vi "SZONE.vi"() -> ()   [LabVIEW 2017]
uses:
  040-typeDefs/Position.ctl
  <vilib>/myRIO/Common/Instrument Driver Framework/myRIO v1.0/Encoder/typedefs/Encoder Signal Mode.ctl
  <vilib>/myRIO/Instrument Drivers/Onboard IO/Encoder/typedefs/Encoder Reference.ctl
  <vilib>/myRIO/Common/Instrument Driver Framework/Utilities/typedefs/myRIO Generic Hardware Reference.ctl
  <vilib>/myRIO/Common/Instrument Driver Framework/Utilities/typedefs/Hardware Version Enum.ctl
  <vilib>/myRIO/Common/Instrument Driver Framework/Utilities/typedefs/myRIO v1.0 Reference.ctl
  <vilib>/myRIO/Common/Instrument Driver Framework/Utilities/typedefs/Generic FPGA Reference.ctl
  <vilib>/myRIO/Common/Instrument Driver Framework/myRIO v1.0/Encoder/typedefs/Encoder Channels Enum.ctl
  <vilib>/myRIO/Common/Instrument Driver Framework/myRIO v1.0/Encoder/typedefs/Encoder Configuration v1.0.ctl
  <vilib>/userdefined/High Color/nirio_resource_hc.ctl
  <vilib>/myRIO/Common/Instrument Driver Framework/Utilities/vis/Is FPGA Ref Available.vi
  <vilib>/myRIO/Common/Instrument Driver Framework/myRIO v1.0/Encoder/vis/myRIO v1.1 Open Encoder.vi
  <vilib>/myRIO/Instrument Drivers/Onboard IO/Encoder/vis/Read.vi
  <vilib>/myRIO/Common/Instrument Driver Framework/Utilities/vis/Validate Channels.vi
  <vilib>/myRIO/Common/Instrument Driver Framework/myRIO v1.0/Encoder/vis/myRIO v1.0 Reserve Encoder.vi
  <vilib>/myRIO/Common/Instrument Driver Framework/myRIO v1.0/Encoder/vis/myRIO v1.0 Build MUX Configuration Encoder.vi
  <vilib>/myRIO/Common/Instrument Driver Framework/myRIO v1.0/Resource Manager/vis/myRIO v1.0 Reserve Channel List.vi
  <vilib>/myRIO/Common/Instrument Driver Framework/myRIO v1.0/Resource Manager/vis/myRIO v1.0 Create Configuration List.vi
  <vilib>/myRIO/Common/Instrument Driver Framework/myRIO v1.0/Resource Manager/vis/myRIO v1.0 Reserve Channel.vi
  <vilib>/myRIO/Common/Instrument Driver Framework/myRIO v1.0/Resource Manager/vis/myRIO v1.0 Unreserve Channel.vi
  <vilib>/myRIO/Common/Instrument Driver Framework/myRIO v1.0/Resource Manager/vis/myRIO v1.0 Build Mutex Name.vi
  <vilib>/Utility/VariantDataType/GetNumericInfo.vi
  <vilib>/Utility/error.llb/Error Cluster From Error Code.vi
  <vilib>/myRIO/Common/Instrument Driver Framework/myRIO v1.0/myRIO v1.1 Open.vi
  <vilib>/myRIO/Common/Instrument Driver Framework/Utilities/vis/IO Manager.vi
  <vilib>/myRIO/Common/Instrument Driver Framework/Utilities/vis/Configuration Manager.vi
  <vilib>/myRIO/Common/Instrument Driver Framework/myRIO v1.0/Resource Manager/vis/myRIO v1.0 Configure IO.vi
  <vilib>/myRIO/Common/Instrument Driver Framework/myRIO v1.0/myRIO v1.0 Close.vi
  <vilib>/myRIO/Common/Instrument Driver Framework/myRIO v1.0/Encoder/vis/myRIO v1.0 Configure Encoder.vi
  <vilib>/myRIO/Common/Instrument Driver Framework/myRIO v1.0/Encoder/vis/myRIO v1.0 Read Encoder.vi
  <vilib>/addons/control/pid/pid.llb/PID (DBL).vi
  <vilib>/myRIO/Express VI/Onboard IO/Encoder/Encoder Express VI.xnode
  <vilib>/myRIO/Instrument Drivers/Onboard IO/Encoder/vis/myRIO Encoder Open.xnode
  <vilib>/myRIO/Common/Instrument Driver Framework/myRIO v1.0/Encoder/typedefs/Encoder Count Direction Enum.ctl
  <vilib>/addons/control/pid/NI_PID_pid.lvlib
  <vilib>/myRIO/Instrument Drivers/Onboard IO/Encoder/Encoder.lvlib
panel:
  in  "Array 5":T1[](array[typedef])=[{"X Pos"=0.0, "Y Pos"=600.0, "Bearing"=0.0}]
  out "Setpoint B 5":dbl(slide)=2.6362825367881695 scale=-10.0..10.0
  out "Setpoint A 5":dbl(slide)=-0.6362825367881695 scale=-10.0..10.0
  out "PID B 5":T2(graph)={"Setpoint"=2.6362825367881695, "output"=0.1428270193177578, "dx/dt"=2.2}
  out "PID A 5":T2(graph)={"Setpoint"=-0.6362825367881695, "output"=-0.0025317711853224956, "dx/dt"=0.0}
  out "OUTPUT A 5":dbl(slide) scale=-10.0..10.0
  out "OUTPUT B 5":dbl(slide)=2.2 scale=-10.0..10.0
  in  "stop 5":bool
  in  "PID gains 5":T3={"proportional gain (Kc)"=0.05, "integral time (Ti, min)"=0.05, "derivative time (Td, min)"=0.0} {"derivative time (Td, min)" format="%.3f"; "integral time (Ti, min)" format="%.3f"; "proportional gain (Kc)" format="%.3f"}
  out "XY Graph 5":cluster{"X":dbl, "Y":dbl}[](graph)=[{"X"=4.58646871556769, "Y"=591.0475853292933}, {"X"=4.6524580319359865, "Y"=591.6424095228513}]
  out "PID Angle 5":cluster{"Bearing":dbl, dbl}(graph)={"Bearing"=-29.103573934109825, 6.330461538461682}
  in  "threshold 5":dbl=10.0
  in  "Max Speed 5":dbl=3.0
  in  "Min Speed 5":dbl=1.0
  out "Final X, Y, BEARING 2":cluster{dbl, dbl, dbl}={4.6524580319359865, 591.6424095228513, 6.330461538461682}
  in  "Array 4":T1[](array[typedef])=[{"X Pos"=0.0, "Y Pos"=400.0, "Bearing"=0.0}]
  out "Setpoint B 4":dbl(slide)=-0.8927738654788293 scale=-10.0..10.0
  out "Setpoint A 4":dbl(slide)=2.892773865478829 scale=-10.0..10.0
  out "PID B 4":T2(graph)={"Setpoint"=-0.8927738654788293, "output"=-0.02661516707895155, "dx/dt"=0.25}
  out "PID A 4":T2(graph)={"Setpoint"=2.892773865478829, "output"=0.16937771953511035, "dx/dt"=1.8520000000000039}
  out "OUTPUT A 4":dbl(slide)=1.8520000000000039 scale=-10.0..10.0
  out "OUTPUT B 4":dbl(slide)=0.25 scale=-10.0..10.0
  in  "stop 4":bool
  in  "PID gains 4":T3={"proportional gain (Kc)"=0.05, "integral time (Ti, min)"=0.05, "derivative time (Td, min)"=0.0} {"derivative time (Td, min)" format="%.3f"; "integral time (Ti, min)" format="%.3f"; "proportional gain (Kc)" format="%.3f"}
  out "XY Graph 4":cluster{"X":dbl, "Y":dbl}[](graph)=[{"X"=1.8269883604661505, "Y"=389.9920566702926}, {"X"=1.4195755255413918, "Y"=390.27970964542567}]
  out "PID Angle 4":cluster{"Bearing":dbl, dbl}(graph)={"Bearing"=-8.308879541892331, -54.77607692307679}
  out "X, Y, BEARING 5":cluster{dbl, dbl, dbl}={1.8269883604661505, 389.9920566702926, -55.01053846153833}
  in  "threshold 4":dbl=10.0
  in  "Max Speed 4":dbl=3.0
  in  "Min Speed 4":dbl=1.0
  in  "Array 3":T1[](array[typedef])=[{"X Pos"=50.0, "Y Pos"=300.0, "Bearing"=0.0}]
  out "Setpoint B 3":dbl(slide)=4.472452663359389 scale=-10.0..10.0
  out "Setpoint A 3":dbl(slide)=-2.4724526633593893 scale=-10.0..10.0
  out "PID B 3":T2(graph)={"Setpoint"=4.472452663359389, "output"=0.25941571832624116, "dx/dt"=2.6666666666666665}
  out "PID A 3":T2(graph)={"Setpoint"=-2.4724526633593893, "output"=-0.12167374508156988, "dx/dt"=-0.617333333333363}
  out "OUTPUT A 3":dbl(slide)=-0.617333333333363 scale=-10.0..10.0
  out "OUTPUT B 3":dbl(slide)=2.6666666666666665 scale=-10.0..10.0
  in  "stop 3":bool
  in  "PID gains 3":T3={"proportional gain (Kc)"=0.05, "integral time (Ti, min)"=0.05, "derivative time (Td, min)"=0.0} {"derivative time (Td, min)" format="%.3f"; "integral time (Ti, min)" format="%.3f"; "proportional gain (Kc)" format="%.3f"}
  out "XY Graph 3":cluster{"X":dbl, "Y":dbl}[](graph)=[{"X"=51.50197299547876, "Y"=290.05042940786}, {"X"=52.04283133633413, "Y"=290.306637655666}]
  out "PID Angle 3":cluster{"Bearing":dbl, dbl}(graph)={"Bearing"=-11.90067630737299, 64.65276923076935}
  out "X, Y, BEARING 4":cluster{dbl, dbl, dbl}={51.50197299547876, 290.05042940786, 65.2389230769232}
  in  "threshold 3":dbl=10.0
  in  "Max Speed 3":dbl=3.0
  in  "Min Speed 3":dbl=1.0
  out "Final X, Y, BEARING 3":cluster{dbl, dbl, dbl}={52.04283133633413, 290.306637655666, 64.65276923076935}
  in  "Array 2":T1[](array[typedef])=[{"X Pos"=-50.0, "Y Pos"=200.0, "Bearing"=0.0}]
  out "Setpoint B 2":dbl(slide)=-1.015688327057204 scale=-10.0..10.0
  out "Setpoint A 2":dbl(slide)=3.015688327057204 scale=-10.0..10.0
  out "PID B 2":T2(graph)={"Setpoint"=-1.015688327057204, "output"=-0.029047263301404516, "dx/dt"=0.0}
  out "PID A 2":T2(graph)={"Setpoint"=3.015688327057204, "output"=0.17494784648736927, "dx/dt"=2.0372000000000012}
  out "OUTPUT A 2":dbl(slide)=2.0372000000000012 scale=-10.0..10.0
  out "OUTPUT B 2":dbl(slide) scale=-10.0..10.0
  in  "stop 2":bool
  in  "PID gains 2":T3={"proportional gain (Kc)"=0.05, "integral time (Ti, min)"=0.05, "derivative time (Td, min)"=0.0} {"derivative time (Td, min)" format="%.3f"; "integral time (Ti, min)" format="%.3f"; "proportional gain (Kc)" format="%.3f"}
  out "XY Graph 2":cluster{"X":dbl, "Y":dbl}[](graph)=[{"X"=-46.776161789477904, "Y"=190.23411508966225}, {"X"=-47.2659069619301, "Y"=190.48132411696224}]
  out "PID Angle 2":cluster{"Bearing":dbl, dbl}(graph)={"Bearing"=-16.02589683272788, -63.216692307692256}
  out "X, Y, BEARING 3":cluster{dbl, dbl, dbl}={-46.776161789477904, 190.23411508966225, -63.53907692307687}
  in  "threshold 2":dbl=10.0
  in  "Max Speed 2":dbl=3.0
  in  "Min Speed 2":dbl=1.0
  in  "Array":T1[](array[typedef])=[{"X Pos"=50.0, "Y Pos"=100.0, "Bearing"=0.0}]
  out "Setpoint B":dbl(slide)=1.38366799687848 scale=-10.0..10.0
  out "Setpoint A":dbl(slide)=0.61633200312152 scale=-10.0..10.0
  out "PID B":T2(graph)={"Setpoint"=1.38366799687848, "output"=0.09818267680403459, "dx/dt"=1.0}
  out "PID A":T2(graph)={"Setpoint"=0.61633200312152, "output"=0.0467575940181558, "dx/dt"=1.1111999999999624}
  out "OUTPUT A":dbl(slide)=1.1111999999999624 scale=-10.0..10.0
  out "OUTPUT B":dbl(slide)=1.0 scale=-10.0..10.0
  in  "stop":bool
  in  "PID gains":T3={"proportional gain (Kc)"=0.05, "integral time (Ti, min)"=0.05, "derivative time (Td, min)"=0.0} {"derivative time (Td, min)" format="%.3f"; "integral time (Ti, min)" format="%.3f"; "proportional gain (Kc)" format="%.3f"}
  out "XY Graph":cluster{"X":dbl, "Y":dbl}[](graph)=[{"X"=44.78345806896074, "Y"=90.79679866901255}, {"X"=45.16607487440638, "Y"=91.25698862034483}]
  out "PID Angle":cluster{"Bearing":dbl, dbl}(graph)={"Bearing"=28.937774880309213, 39.74123076923079}
  out "X, Y, BEARING 2":cluster{dbl, dbl, dbl}={44.78345806896074, 90.79679866901255, 39.74123076923079}
  in  "threshold":dbl=10.0
  in  "Max Speed":dbl=3.0
  in  "Min Speed":dbl=1.0
  in  "Initial X, Y, BEARING":cluster{dbl, dbl, dbl}
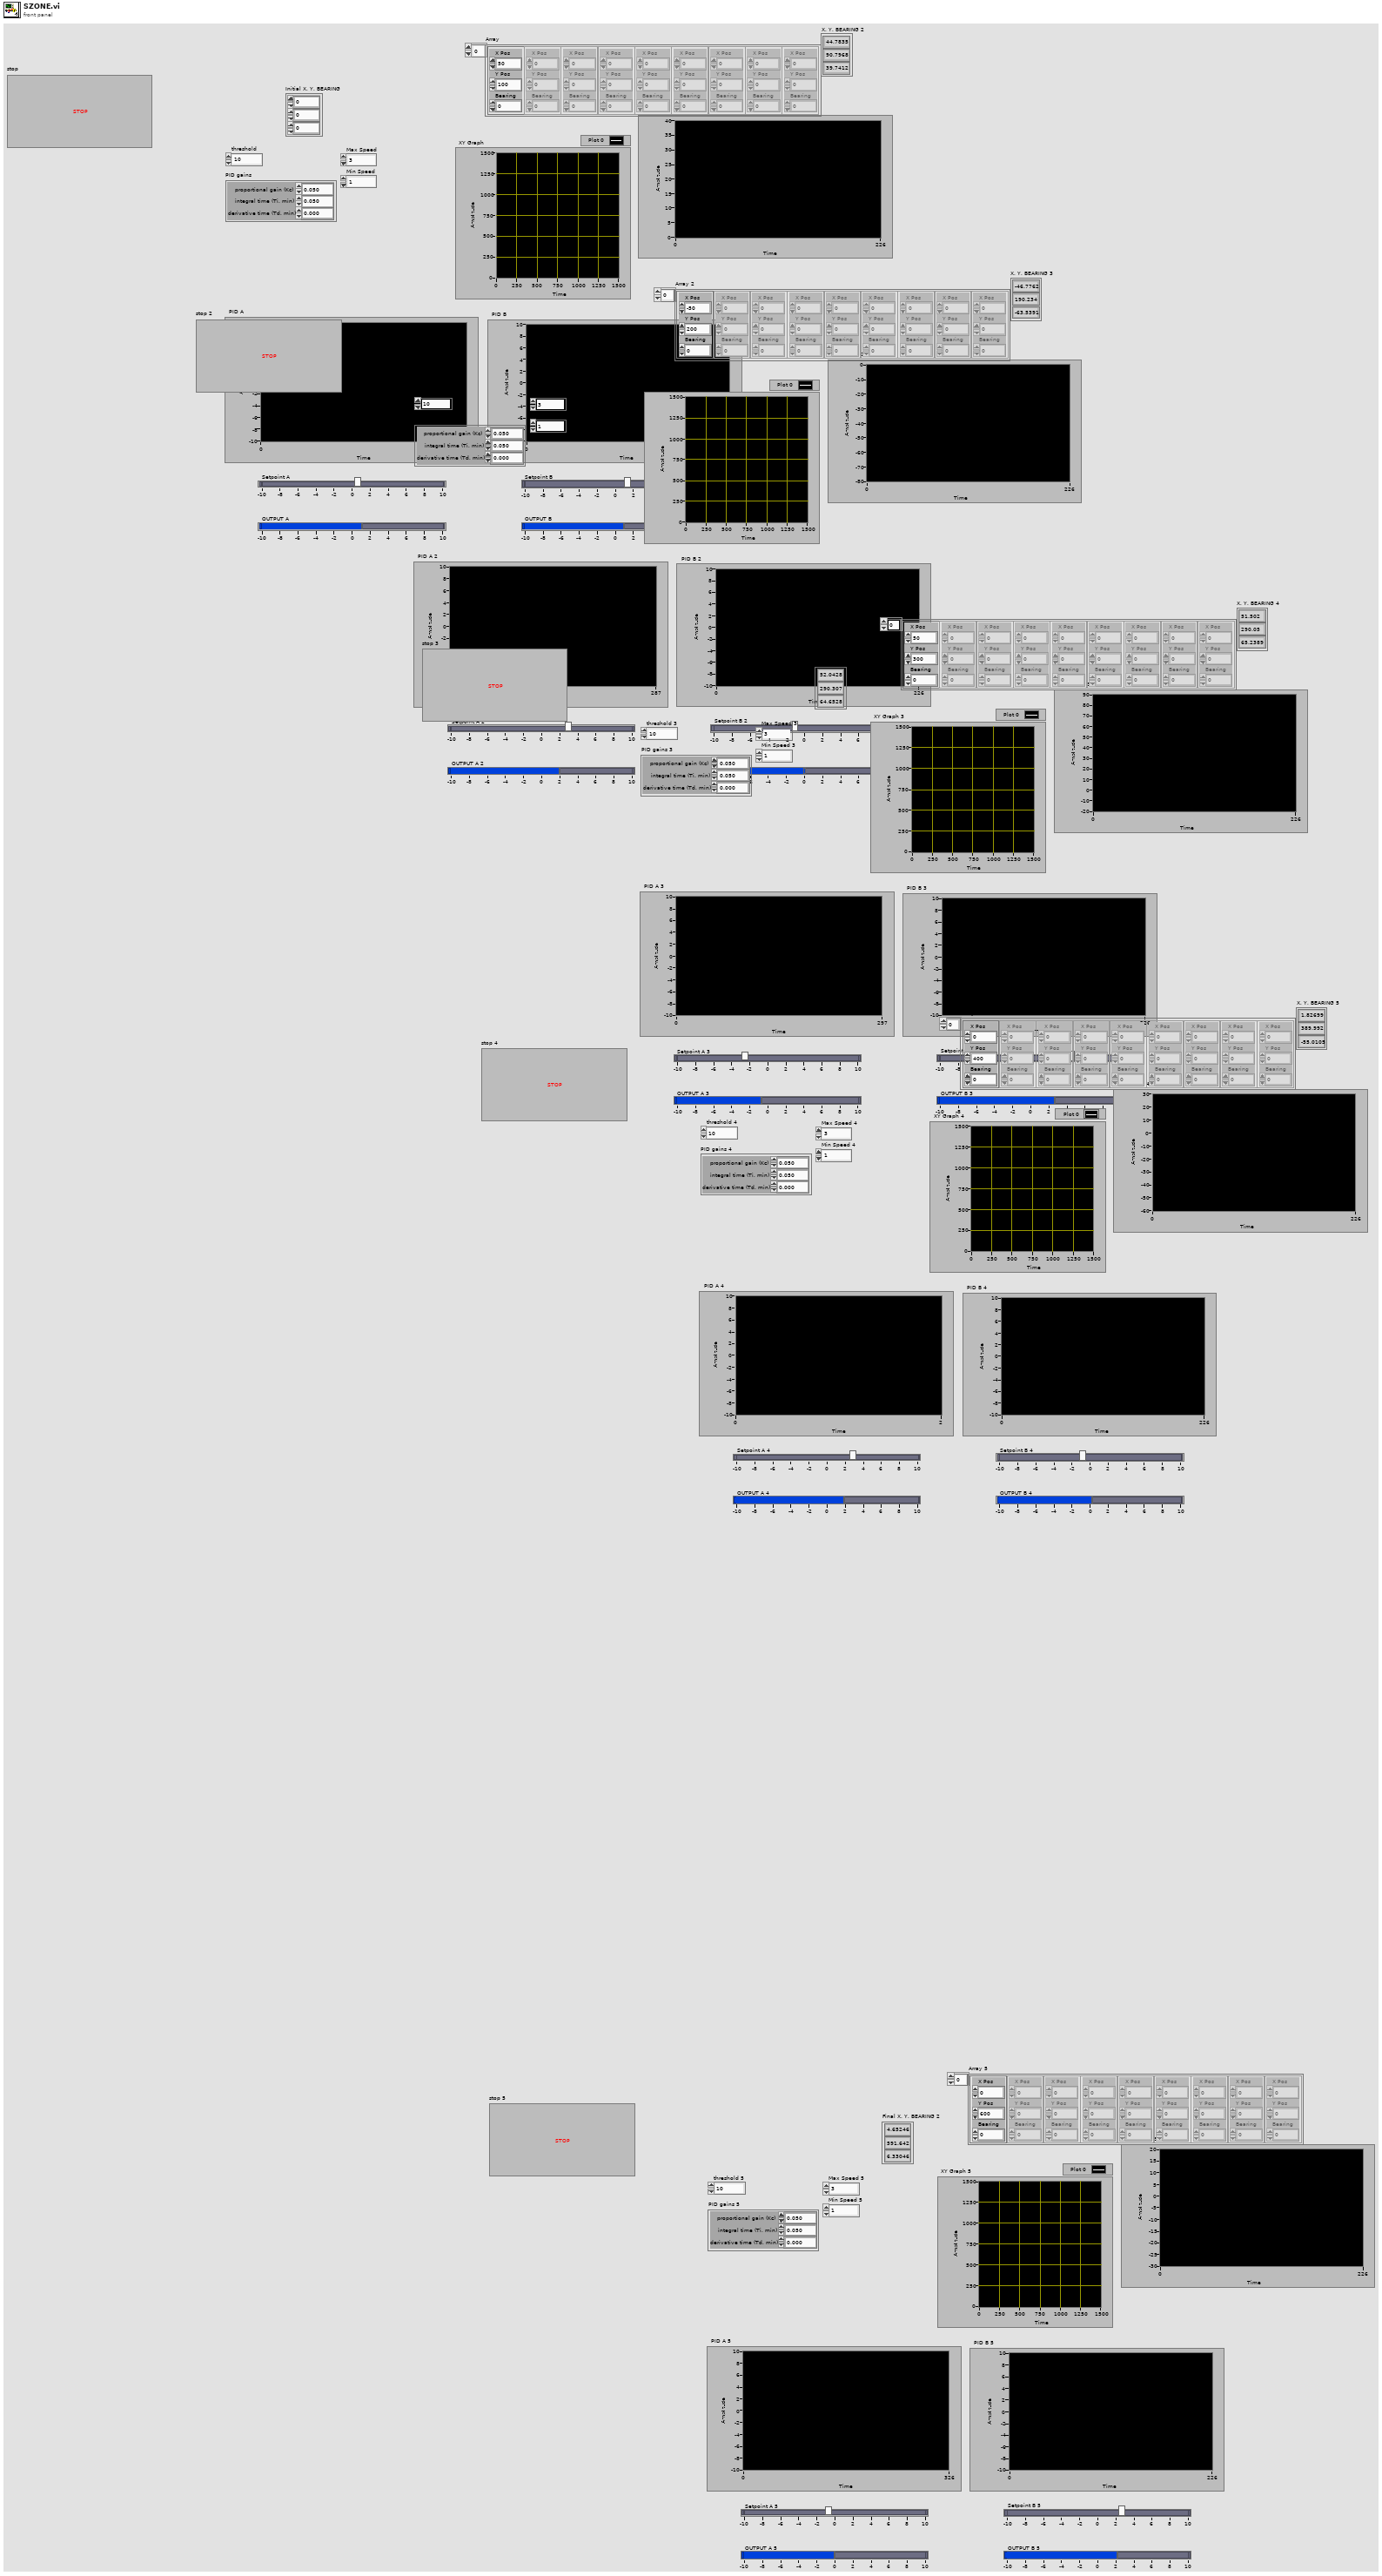
[diagram p1: front panel]
types:
  T1 = typedef "Position.ctl" = cluster{"X Pos":dbl, "Y Pos":dbl, "Bearing":dbl}
  T2 = cluster{"Setpoint":dbl, "output":dbl, "dx/dt":dbl}
  T3 = cluster{"proportional gain (Kc)":dbl, "integral time (Ti, min)":dbl, "derivative time (Td, min)":dbl}
  T4 = typedef "Encoder.lvlib/Encoder Reference.ctl" = cluster{"myRIO Reference":T5, "Encoder Channels Enum":T9}
  T5 = typedef "myRIO Generic Hardware Reference.ctl" = cluster{"myRIO Model":T6, "myRIO Hardware Reference":T7}
  T6 = typedef "Hardware Version Enum.ctl" = enum16{"Unknown", "myRIO-1900", "myRIO-1950", "roboRIO", "NI ELVIS RIO CM"}
  T7 = typedef "myRIO v1.0 Reference.ctl" = cluster{"Generic FPGA Reference":T8, "Allow multiple opens":bool}
  T8 = typedef "Generic FPGA Reference.ctl" = refnum<k20>
  T9 = typedef "Encoder Channels Enum.ctl" = enum16{"Not Connected", "C/ENC0", "C/ENC1", "A/ENC", "B/ENC", "DIO/ENC0", "DIO/ENC1", "DIO/ENC2", "DIO/ENC3", "DIO/ENC4"}
  T10 = typedef "Encoder Signal Mode.ctl" = enum16{"Quadrature phase signal", "Step and direction signal"}
  T11 = typedef "nirio_resource_hc.ctl" = tag
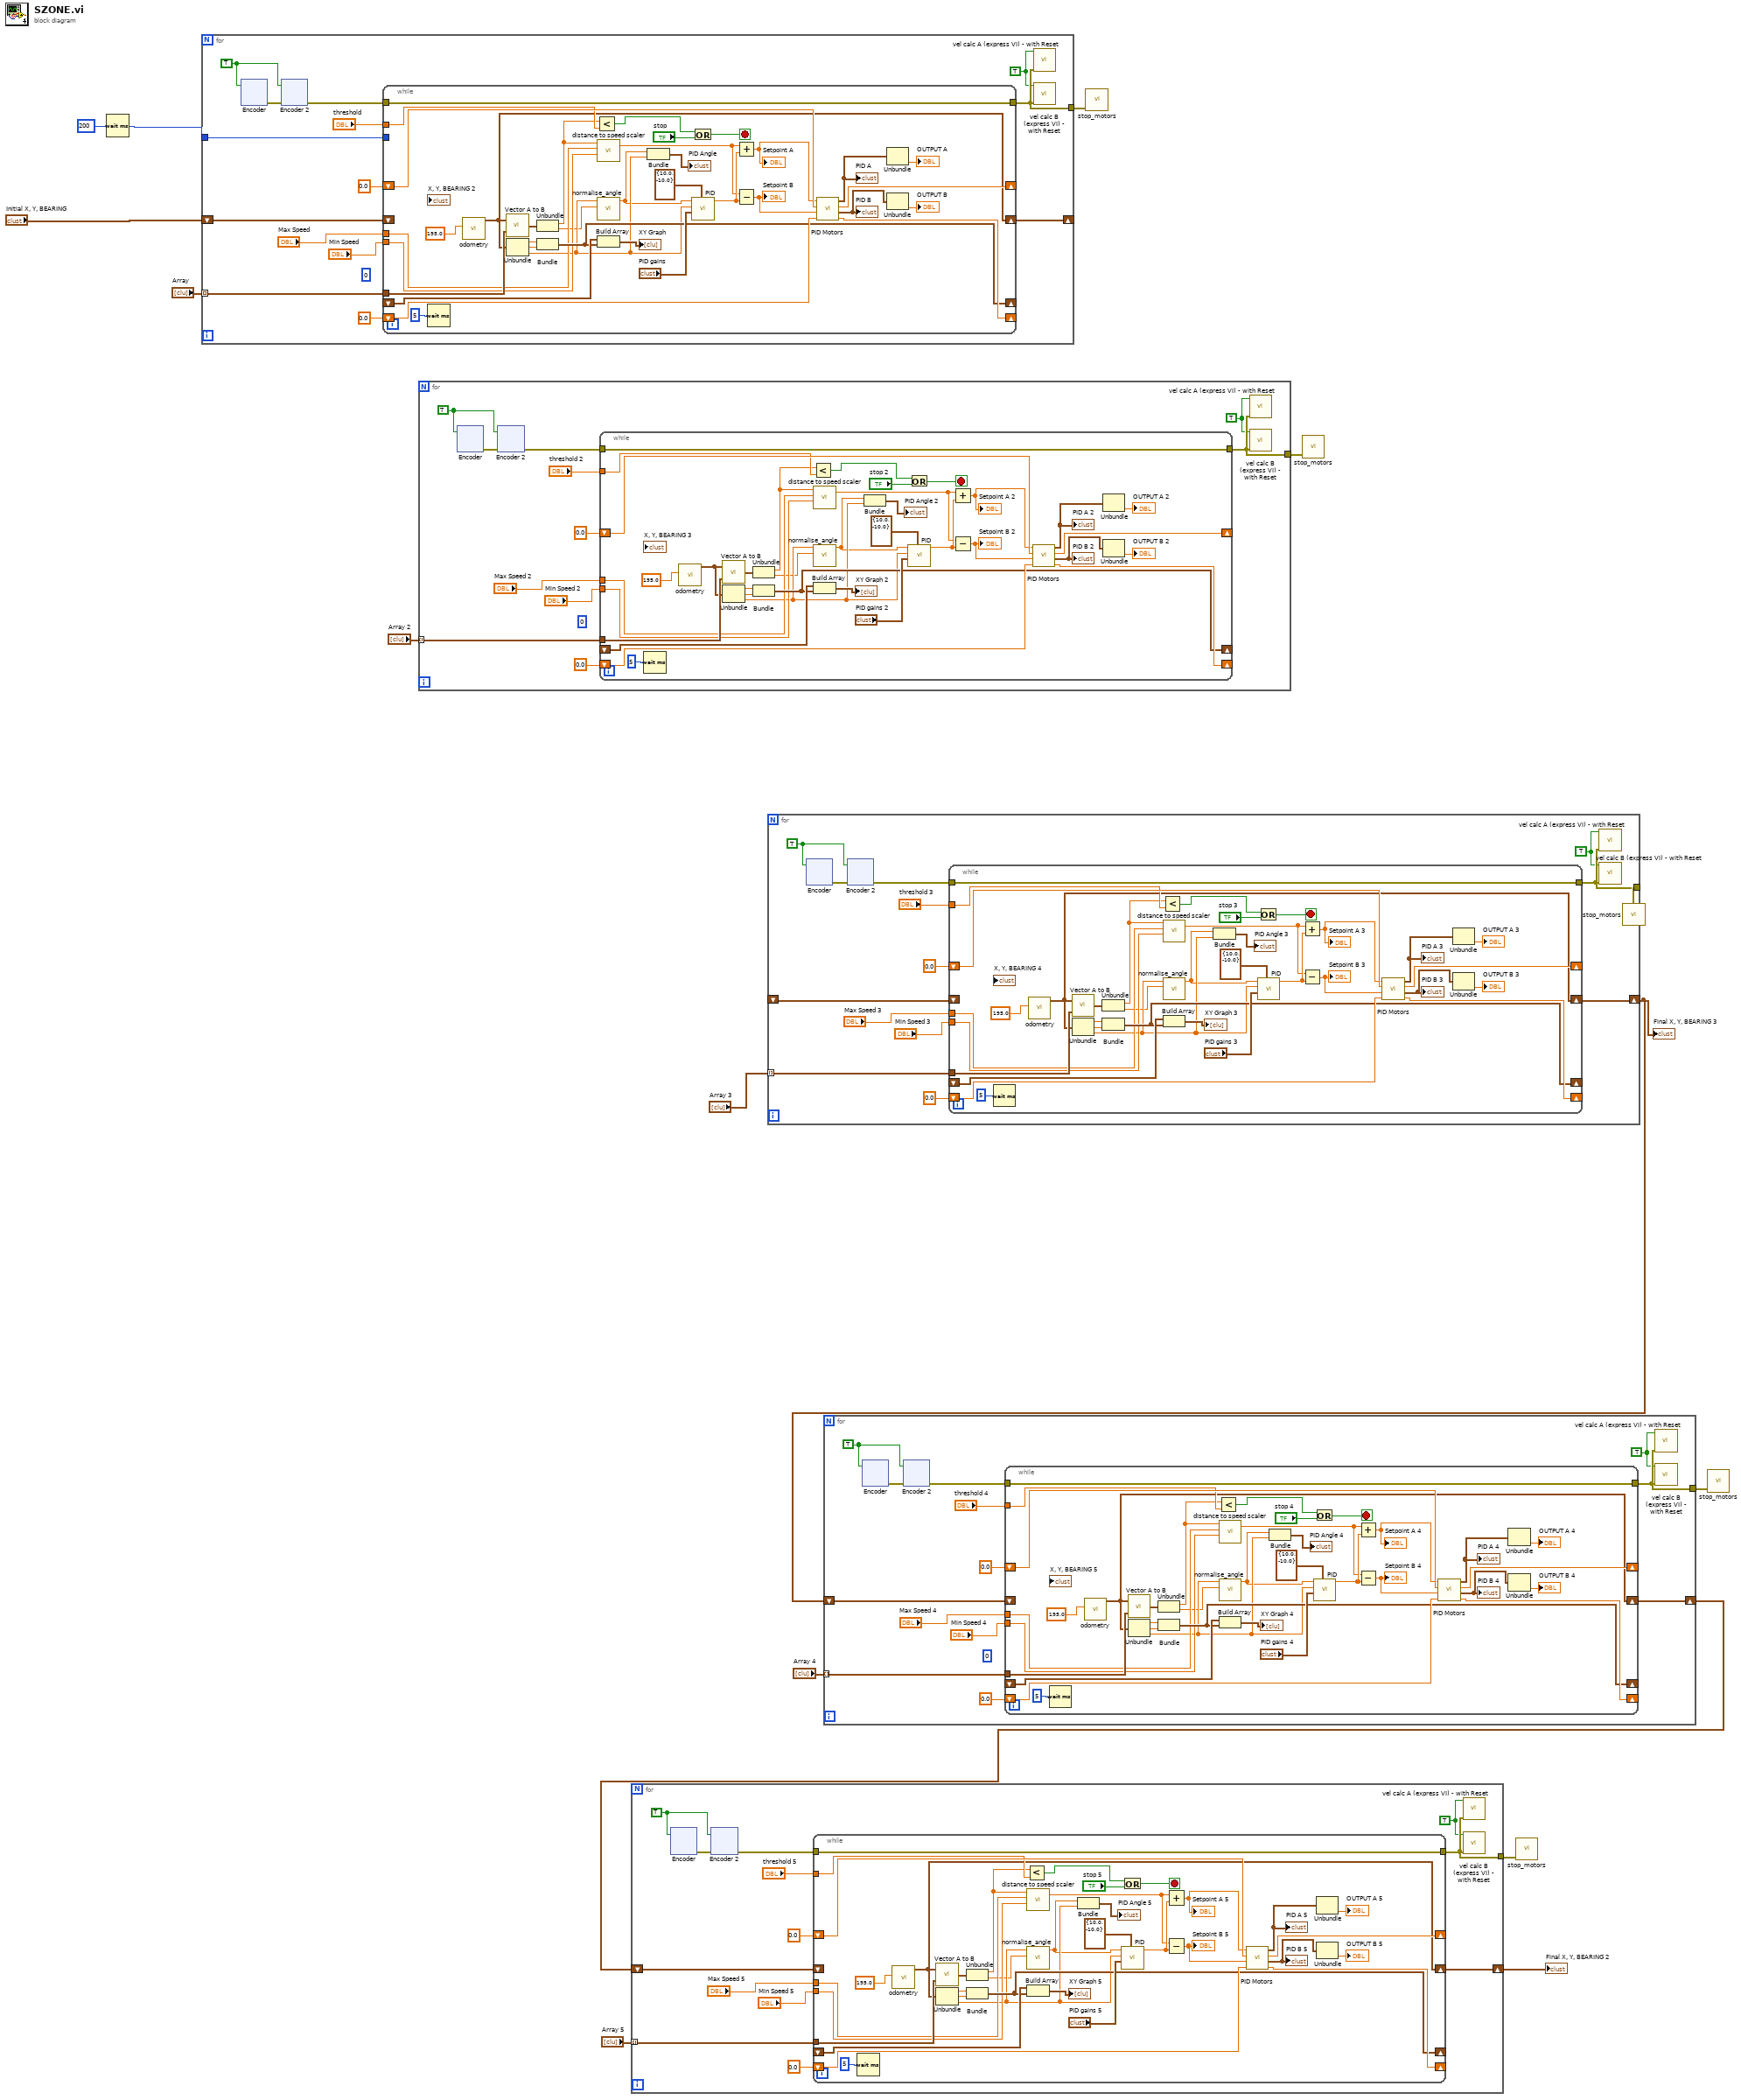
[diagram p0: block diagram]
diagram:
  n1 = Wait (ms)(milliseconds to wait=u32 200) -> (millisecond timer value=w12:u32)
  n2 = for {
    shift-right: [w25] -> _
    shift-left: "Initial X, Y, BEARING" -> [w24]
    tunnel: "Array" -> [w23] mode=indexing
    tunnel: [w19] -> w15
    tunnel: w12 -> [w17]
    w18 = TRUE ("Reinitialise")
    w21 = TRUE
    (unwired) 0 ("ENCA OUT")
    n3 = xnode "Encoder"("Reset Counter"=w21) -> ("error out"=w22:errorcluster)  [unwired: 1 in, 3 out]
    n4 = xnode "Encoder 2"("error in (no error)"=w22, "Reset Counter"=w21) -> ("error out"=w20:errorcluster)  [unwired: 3 out]
    n5 = while {
      tunnel: w20 -> [w152]
      shift-right: [w154] -> _
      shift-left: 0.0 ("output A") -> [w155]
      shift-right: [w157] -> _
      shift-left: 0.0 ("output B") -> [w156]
      tunnel: [w152] -> w19
      tunnel: w23 -> [w143]
      tunnel: "threshold" -> [w139]
      shift-right: [w137] -> w25
      shift-left: w24 -> [_]
      shift-right: [w133] -> _
      shift-left: _ -> [w134]
      tunnel: "Max Speed" -> [w128]
      tunnel: "Min Speed" -> [w127]
      tunnel: w17 -> [_]
      stop <- w140 stop-if-true
      n6 = Wait (ms)(milliseconds to wait=5 ("ENCB OUT")) -> ()  [unwired: 1 out]
      n7 = call "odometry.vi"("wheelbase"=195.0) -> ("X, Y, BEARING"=w137:cluster{dbl, dbl, dbl})  [unwired: 7 in, 2 out]
      n8 = call "Vector A to B.vi"("Destination"=w143, "Current"=w137) -> ("vector"=w142:cluster{dbl, "Bearing":dbl})
      n9 = Unbundle(w137) -> (w135:dbl, w136:dbl, w125:dbl)
      n10 = Unbundle(w142) -> (w129:dbl, "Bearing"=w124:dbl)
      n11 = Bundle(w135, w136) -> (w133:cluster{dbl, dbl})  [unwired: 1 in]
      n12 = Less?(x=w129, y=w139) -> (x < y?=w138:bool)
      n13 = call "distance to speed scaler.vi"("Min Speed"=w127, "Max Speed"=w128, "Distance (mm)"=w129) -> ("Speed (0..10)"=w130:dbl)  [unwired: 2 in]
      n14 = call "normalise_angle.vi"("target -180 .. 180"=w124, "current"=w125) -> ("travel_direction"=w123:dbl)  [unwired: 9 in]
      n15 = Build Array(w134, w133) -> (→"XY Graph":cluster{dbl, dbl}[])
      n16 = Bundle("travel_direction"=w123, w125) -> (→"PID Angle":cluster{"travel_direction":dbl, dbl})  [unwired: 1 in]
      n17 = Or(x=w138, y="stop") -> (x .or. y?=w140:bool)
      n18 = call-poly <vilib>:"PID.vi"("output range"=cluster{"output high":dbl, "output low":dbl} {"output high"=10.0, "output low"=-10.0}, "PID gains"="PID gains", "process variable"=w125, "setpoint"=w123) -> ("output"=w147:dbl)  [unwired: 6 in, 1 out]
      n19 = Add(x=w130, y=w147) -> (x+y=w144:dbl)
      "Setpoint A" <- w144
      n20 = Subtract(x=w130, y=w147) -> (x-y=w145:dbl)
      "Setpoint B" <- w145
      n21 = call "PID Motors.vi"("input B"=w156, "Speed B"=w145, "input A"=w155, "Speed A"=w144) -> ("output B"=w157:dbl, "Speed B0"=w150:T2, "output A"=w154:dbl, "Speed A0"=w151:T2)
      "PID B" <- w150
      "PID A" <- w151
      n22 = Unbundle(w151) -> ("dx/dt"=→"OUTPUT A":dbl)  [unwired: 2 out]
      n23 = Unbundle(w150) -> ("dx/dt"=→"OUTPUT B":dbl)  [unwired: 2 out]
    }
    n24 = call "vel calc A (express VI) - with Reset.vi"("error in"=w19, "Reinitialise"=w18) -> ()  [unwired: 5 in, 5 out]
    n25 = call "vel calc B (express VI) - with Reset.vi"("error in"=w19, "Reinitialise"=w18) -> ()  [unwired: 5 in, 5 out]
  }
  n26 = for {
    tunnel: "Array 2" -> [w164] mode=indexing
    tunnel: [w160] -> w10
    w159 = TRUE ("Reinitialise")
    w162 = TRUE
    (unwired) 0 ("ENCA OUT")
    n27 = xnode "Encoder"("Reset Counter"=w162) -> ("error out"=w163:errorcluster)  [unwired: 1 in, 3 out]
    n28 = xnode "Encoder 2"("error in (no error)"=w163, "Reset Counter"=w162) -> ("error out"=w161:errorcluster)  [unwired: 3 out]
    n29 = while {
      tunnel: w161 -> [w291]
      shift-right: [w293] -> _
      shift-left: 0.0 ("output A") -> [w294]
      shift-right: [w296] -> _
      shift-left: 0.0 ("output B") -> [w295]
      tunnel: [w291] -> w160
      tunnel: w164 -> [w282]
      tunnel: "threshold 2" -> [w278]
      shift-right: [w272] -> _
      shift-left: _ -> [w273]
      tunnel: "Max Speed 2" -> [w267]
      tunnel: "Min Speed 2" -> [w266]
      stop <- w279 stop-if-true
      n30 = Wait (ms)(milliseconds to wait=5 ("ENCB OUT")) -> ()  [unwired: 1 out]
      n31 = call "odometry.vi"("wheelbase"=195.0) -> ("X, Y, BEARING"=w276:cluster{dbl, dbl, dbl})  [unwired: 7 in, 2 out]
      n32 = call "Vector A to B.vi"("Destination"=w282, "Current"=w276) -> ("vector"=w281:cluster{dbl, "Bearing":dbl})
      n33 = Unbundle(w276) -> (w274:dbl, w275:dbl, w264:dbl)
      n34 = Unbundle(w281) -> (w268:dbl, "Bearing"=w263:dbl)
      n35 = Bundle(w274, w275) -> (w272:cluster{dbl, dbl})  [unwired: 1 in]
      n36 = Less?(x=w268, y=w278) -> (x < y?=w277:bool)
      n37 = call "distance to speed scaler.vi"("Min Speed"=w266, "Max Speed"=w267, "Distance (mm)"=w268) -> ("Speed (0..10)"=w269:dbl)  [unwired: 2 in]
      n38 = call "normalise_angle.vi"("target -180 .. 180"=w263, "current"=w264) -> ("travel_direction"=w262:dbl)  [unwired: 9 in]
      n39 = Build Array(w273, w272) -> (→"XY Graph 2":cluster{dbl, dbl}[])
      n40 = Bundle("travel_direction"=w262, w264) -> (→"PID Angle 2":cluster{"travel_direction":dbl, dbl})  [unwired: 1 in]
      n41 = Or(x=w277, y="stop 2") -> (x .or. y?=w279:bool)
      n42 = call-poly <vilib>:"PID.vi"("output range"=cluster{"output high":dbl, "output low":dbl} {"output high"=10.0, "output low"=-10.0}, "PID gains"="PID gains 2", "process variable"=w264, "setpoint"=w262) -> ("output"=w286:dbl)  [unwired: 6 in, 1 out]
      n43 = Add(x=w269, y=w286) -> (x+y=w283:dbl)
      "Setpoint A 2" <- w283
      n44 = Subtract(x=w269, y=w286) -> (x-y=w284:dbl)
      "Setpoint B 2" <- w284
      n45 = call "PID Motors.vi"("input B"=w295, "Speed B"=w284, "input A"=w294, "Speed A"=w283) -> ("output B"=w296:dbl, "Speed B0"=w289:T2, "output A"=w293:dbl, "Speed A0"=w290:T2)
      "PID B 2" <- w289
      "PID A 2" <- w290
      n46 = Unbundle(w290) -> ("dx/dt"=→"OUTPUT A 2":dbl)  [unwired: 2 out]
      n47 = Unbundle(w289) -> ("dx/dt"=→"OUTPUT B 2":dbl)  [unwired: 2 out]
    }
    n48 = call "vel calc A (express VI) - with Reset.vi"("error in"=w160, "Reinitialise"=w159) -> ()  [unwired: 5 in, 5 out]
    n49 = call "vel calc B (express VI) - with Reset.vi"("error in"=w160, "Reinitialise"=w159) -> ()  [unwired: 5 in, 5 out]
  }
  n50 = for {
    shift-right: [w305] -> w5
    shift-left: _ -> [w304]
    tunnel: "Array 3" -> [w303] mode=indexing
    tunnel: [w299] -> w8
    w298 = TRUE ("Reinitialise")
    w301 = TRUE
    n51 = xnode "Encoder"("Reset Counter"=w301) -> ("error out"=w302:errorcluster)  [unwired: 1 in, 3 out]
    n52 = xnode "Encoder 2"("error in (no error)"=w302, "Reset Counter"=w301) -> ("error out"=w300:errorcluster)  [unwired: 3 out]
    n53 = while {
      tunnel: w300 -> [w432]
      shift-right: [w434] -> _
      shift-left: 0.0 ("output A") -> [w435]
      shift-right: [w437] -> _
      shift-left: 0.0 ("output B") -> [w436]
      tunnel: [w432] -> w299
      tunnel: w303 -> [w423]
      tunnel: "threshold 3" -> [w419]
      shift-right: [w417] -> w305
      shift-left: w304 -> [_]
      shift-right: [w413] -> _
      shift-left: _ -> [w414]
      tunnel: "Max Speed 3" -> [w408]
      tunnel: "Min Speed 3" -> [w407]
      stop <- w420 stop-if-true
      n54 = Wait (ms)(milliseconds to wait=5 ("ENCB OUT")) -> ()  [unwired: 1 out]
      n55 = call "odometry.vi"("wheelbase"=195.0) -> ("X, Y, BEARING"=w417:cluster{dbl, dbl, dbl})  [unwired: 7 in, 2 out]
      n56 = call "Vector A to B.vi"("Destination"=w423, "Current"=w417) -> ("vector"=w422:cluster{dbl, "Bearing":dbl})
      n57 = Unbundle(w417) -> (w415:dbl, w416:dbl, w405:dbl)
      n58 = Unbundle(w422) -> (w409:dbl, "Bearing"=w404:dbl)
      n59 = Bundle(w415, w416) -> (w413:cluster{dbl, dbl})  [unwired: 1 in]
      n60 = Less?(x=w409, y=w419) -> (x < y?=w418:bool)
      n61 = call "distance to speed scaler.vi"("Min Speed"=w407, "Max Speed"=w408, "Distance (mm)"=w409) -> ("Speed (0..10)"=w410:dbl)  [unwired: 2 in]
      n62 = call "normalise_angle.vi"("target -180 .. 180"=w404, "current"=w405) -> ("travel_direction"=w403:dbl)  [unwired: 9 in]
      n63 = Build Array(w414, w413) -> (→"XY Graph 3":cluster{dbl, dbl}[])
      n64 = Bundle("travel_direction"=w403, w405) -> (→"PID Angle 3":cluster{"travel_direction":dbl, dbl})  [unwired: 1 in]
      n65 = Or(x=w418, y="stop 3") -> (x .or. y?=w420:bool)
      n66 = call-poly <vilib>:"PID.vi"("output range"=cluster{"output high":dbl, "output low":dbl} {"output high"=10.0, "output low"=-10.0}, "PID gains"="PID gains 3", "process variable"=w405, "setpoint"=w403) -> ("output"=w427:dbl)  [unwired: 6 in, 1 out]
      n67 = Add(x=w410, y=w427) -> (x+y=w424:dbl)
      "Setpoint A 3" <- w424
      n68 = Subtract(x=w410, y=w427) -> (x-y=w425:dbl)
      "Setpoint B 3" <- w425
      n69 = call "PID Motors.vi"("input B"=w436, "Speed B"=w425, "input A"=w435, "Speed A"=w424) -> ("output B"=w437:dbl, "Speed B0"=w430:T2, "output A"=w434:dbl, "Speed A0"=w431:T2)
      "PID B 3" <- w430
      "PID A 3" <- w431
      n70 = Unbundle(w431) -> ("dx/dt"=→"OUTPUT A 3":dbl)  [unwired: 2 out]
      n71 = Unbundle(w430) -> ("dx/dt"=→"OUTPUT B 3":dbl)  [unwired: 2 out]
    }
    n72 = call "vel calc A (express VI) - with Reset.vi"("error in"=w299, "Reinitialise"=w298) -> ()  [unwired: 5 in, 5 out]
    n73 = call "vel calc B (express VI) - with Reset.vi"("error in"=w299, "Reinitialise"=w298) -> ()  [unwired: 5 in, 5 out]
  }
  "Final X, Y, BEARING 3" <- w5
  n74 = for {
    shift-right: [w446] -> w1
    shift-left: w5 -> [w445]
    tunnel: "Array 4" -> [w444] mode=indexing
    tunnel: [w440] -> w6
    w439 = TRUE ("Reinitialise")
    w442 = TRUE
    (unwired) 0 ("ENCA OUT")
    n75 = xnode "Encoder"("Reset Counter"=w442) -> ("error out"=w443:errorcluster)  [unwired: 1 in, 3 out]
    n76 = xnode "Encoder 2"("error in (no error)"=w443, "Reset Counter"=w442) -> ("error out"=w441:errorcluster)  [unwired: 3 out]
    n77 = while {
      tunnel: w441 -> [w573]
      shift-right: [w575] -> _
      shift-left: 0.0 ("output A") -> [w576]
      shift-right: [w578] -> _
      shift-left: 0.0 ("output B") -> [w577]
      tunnel: [w573] -> w440
      tunnel: w444 -> [w564]
      tunnel: "threshold 4" -> [w560]
      shift-right: [w558] -> w446
      shift-left: w445 -> [_]
      shift-right: [w554] -> _
      shift-left: _ -> [w555]
      tunnel: "Max Speed 4" -> [w549]
      tunnel: "Min Speed 4" -> [w548]
      stop <- w561 stop-if-true
      n78 = Wait (ms)(milliseconds to wait=5 ("ENCB OUT")) -> ()  [unwired: 1 out]
      n79 = call "odometry.vi"("wheelbase"=195.0) -> ("X, Y, BEARING"=w558:cluster{dbl, dbl, dbl})  [unwired: 7 in, 2 out]
      n80 = call "Vector A to B.vi"("Destination"=w564, "Current"=w558) -> ("vector"=w563:cluster{dbl, "Bearing":dbl})
      n81 = Unbundle(w558) -> (w556:dbl, w557:dbl, w546:dbl)
      n82 = Unbundle(w563) -> (w550:dbl, "Bearing"=w545:dbl)
      n83 = Bundle(w556, w557) -> (w554:cluster{dbl, dbl})  [unwired: 1 in]
      n84 = Less?(x=w550, y=w560) -> (x < y?=w559:bool)
      n85 = call "distance to speed scaler.vi"("Min Speed"=w548, "Max Speed"=w549, "Distance (mm)"=w550) -> ("Speed (0..10)"=w551:dbl)  [unwired: 2 in]
      n86 = call "normalise_angle.vi"("target -180 .. 180"=w545, "current"=w546) -> ("travel_direction"=w544:dbl)  [unwired: 9 in]
      n87 = Build Array(w555, w554) -> (→"XY Graph 4":cluster{dbl, dbl}[])
      n88 = Bundle("travel_direction"=w544, w546) -> (→"PID Angle 4":cluster{"travel_direction":dbl, dbl})  [unwired: 1 in]
      n89 = Or(x=w559, y="stop 4") -> (x .or. y?=w561:bool)
      n90 = call-poly <vilib>:"PID.vi"("output range"=cluster{"output high":dbl, "output low":dbl} {"output high"=10.0, "output low"=-10.0}, "PID gains"="PID gains 4", "process variable"=w546, "setpoint"=w544) -> ("output"=w568:dbl)  [unwired: 6 in, 1 out]
      n91 = Add(x=w551, y=w568) -> (x+y=w565:dbl)
      "Setpoint A 4" <- w565
      n92 = Subtract(x=w551, y=w568) -> (x-y=w566:dbl)
      "Setpoint B 4" <- w566
      n93 = call "PID Motors.vi"("input B"=w577, "Speed B"=w566, "input A"=w576, "Speed A"=w565) -> ("output B"=w578:dbl, "Speed B0"=w571:T2, "output A"=w575:dbl, "Speed A0"=w572:T2)
      "PID B 4" <- w571
      "PID A 4" <- w572
      n94 = Unbundle(w572) -> ("dx/dt"=→"OUTPUT A 4":dbl)  [unwired: 2 out]
      n95 = Unbundle(w571) -> ("dx/dt"=→"OUTPUT B 4":dbl)  [unwired: 2 out]
    }
    n96 = call "vel calc A (express VI) - with Reset.vi"("error in"=w440, "Reinitialise"=w439) -> ()  [unwired: 5 in, 5 out]
    n97 = call "vel calc B (express VI) - with Reset.vi"("error in"=w440, "Reinitialise"=w439) -> ()  [unwired: 5 in, 5 out]
  }
  n98 = for {
    shift-right: [w587] -> w4
    shift-left: w1 -> [w586]
    tunnel: "Array 5" -> [w585] mode=indexing
    tunnel: [w581] -> w2
    w580 = TRUE ("Reinitialise")
    w583 = TRUE
    n99 = xnode "Encoder"("Reset Counter"=w583) -> ("error out"=w584:errorcluster)  [unwired: 1 in, 3 out]
    n100 = xnode "Encoder 2"("error in (no error)"=w584, "Reset Counter"=w583) -> ("error out"=w582:errorcluster)  [unwired: 3 out]
    n101 = while {
      tunnel: w582 -> [w714]
      shift-right: [w716] -> _
      shift-left: 0.0 ("output A") -> [w717]
      shift-right: [w719] -> _
      shift-left: 0.0 ("output B") -> [w718]
      tunnel: [w714] -> w581
      tunnel: w585 -> [w705]
      tunnel: "threshold 5" -> [w701]
      shift-right: [w699] -> w587
      shift-left: w586 -> [_]
      shift-right: [w695] -> _
      shift-left: _ -> [w696]
      tunnel: "Max Speed 5" -> [w690]
      tunnel: "Min Speed 5" -> [w689]
      stop <- w702 stop-if-true
      n102 = Wait (ms)(milliseconds to wait=5 ("ENCB OUT")) -> ()  [unwired: 1 out]
      n103 = call "odometry.vi"("wheelbase"=195.0) -> ("X, Y, BEARING"=w699:cluster{dbl, dbl, dbl})  [unwired: 7 in, 2 out]
      n104 = call "Vector A to B.vi"("Destination"=w705, "Current"=w699) -> ("vector"=w704:cluster{dbl, "Bearing":dbl})
      n105 = Unbundle(w699) -> (w697:dbl, w698:dbl, w687:dbl)
      n106 = Unbundle(w704) -> (w691:dbl, "Bearing"=w686:dbl)
      n107 = Bundle(w697, w698) -> (w695:cluster{dbl, dbl})  [unwired: 1 in]
      n108 = Less?(x=w691, y=w701) -> (x < y?=w700:bool)
      n109 = call "distance to speed scaler.vi"("Min Speed"=w689, "Max Speed"=w690, "Distance (mm)"=w691) -> ("Speed (0..10)"=w692:dbl)  [unwired: 2 in]
      n110 = call "normalise_angle.vi"("target -180 .. 180"=w686, "current"=w687) -> ("travel_direction"=w685:dbl)  [unwired: 9 in]
      n111 = Build Array(w696, w695) -> (→"XY Graph 5":cluster{dbl, dbl}[])
      n112 = Bundle("travel_direction"=w685, w687) -> (→"PID Angle 5":cluster{"travel_direction":dbl, dbl})  [unwired: 1 in]
      n113 = Or(x=w700, y="stop 5") -> (x .or. y?=w702:bool)
      n114 = call-poly <vilib>:"PID.vi"("output range"=cluster{"output high":dbl, "output low":dbl} {"output high"=10.0, "output low"=-10.0}, "PID gains"="PID gains 5", "process variable"=w687, "setpoint"=w685) -> ("output"=w709:dbl)  [unwired: 6 in, 1 out]
      n115 = Add(x=w692, y=w709) -> (x+y=w706:dbl)
      "Setpoint A 5" <- w706
      n116 = Subtract(x=w692, y=w709) -> (x-y=w707:dbl)
      "Setpoint B 5" <- w707
      n117 = call "PID Motors.vi"("input B"=w718, "Speed B"=w707, "input A"=w717, "Speed A"=w706) -> ("output B"=w719:dbl, "Speed B0"=w712:T2, "output A"=w716:dbl, "Speed A0"=w713:T2)
      "PID B 5" <- w712
      "PID A 5" <- w713
      n118 = Unbundle(w713) -> ("dx/dt"=→"OUTPUT A 5":dbl)  [unwired: 2 out]
      n119 = Unbundle(w712) -> ("dx/dt"=→"OUTPUT B 5":dbl)  [unwired: 2 out]
    }
    n120 = call "vel calc A (express VI) - with Reset.vi"("error in"=w581, "Reinitialise"=w580) -> ()  [unwired: 5 in, 5 out]
    n121 = call "vel calc B (express VI) - with Reset.vi"("error in"=w581, "Reinitialise"=w580) -> ()  [unwired: 5 in, 5 out]
  }
  "Final X, Y, BEARING 2" <- w4
  n122 = call "stop_motors.vi"("error in (no error)"=w15) -> ()  [unwired: 4 in, 1 out]
  n123 = call "stop_motors.vi"("error in (no error)"=w10) -> ()  [unwired: 4 in, 1 out]
  n124 = call "stop_motors.vi"("error in (no error)"=w2) -> ()  [unwired: 4 in, 1 out]
  n125 = call "stop_motors.vi"("error in (no error)"=w8) -> ()  [unwired: 4 in, 1 out]
  n126 = call "stop_motors.vi"("error in (no error)"=w6) -> ()  [unwired: 4 in, 1 out]
